vi "error subvi.vi"(0 "error out":errorcluster) -> ()   [LabVIEW 2009]
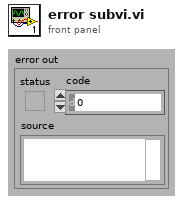
[diagram p1: front panel]
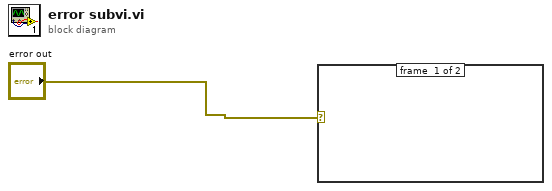
[diagram p0: block diagram]
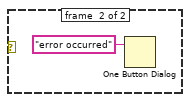
[diagram p2: hidden frame]
diagram:
  n1 = case shown="Error" "error out" {
    frame #0 {
    }
    frame #1 {
      n2 = One Button Dialog(message="error occurred") -> ()  [unwired: 1 in, 1 out]
    }
  }
